vi "Count Event Message by Message.vi"(8 "error in (no error)":errorcluster, 9 "Timeout":i32, 10 "Message":string, 11 "Event Registration Refnum in":refnum<event-registration>) -> (0 "error out":errorcluster, 1 "Message Data":variant[](array[variant]), 2 "Count":i32, 3 "Event Registration Refnum out":refnum<event-registration>)   [LabVIEW 2020, in "Framework Test Support.lvlib" / "Event Helpers.lvlib"]
uses:
  Event Helpers.lvlib
  Framework/Process/Protected/Broadcasting/Broadcast Message Cluster.ctl
  Execution timer.vi
  Dequeue Event Message.vi
  Framework/Process/Process.lvclass
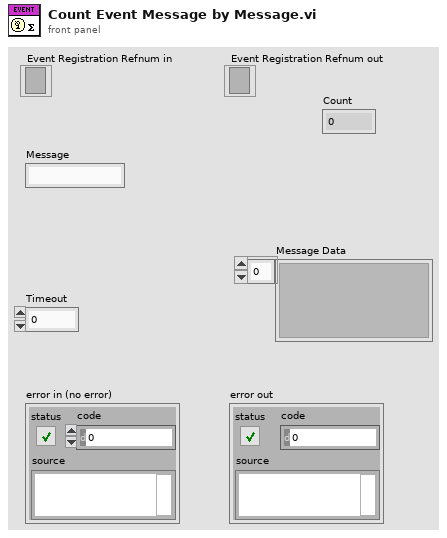
[diagram p1: front panel]
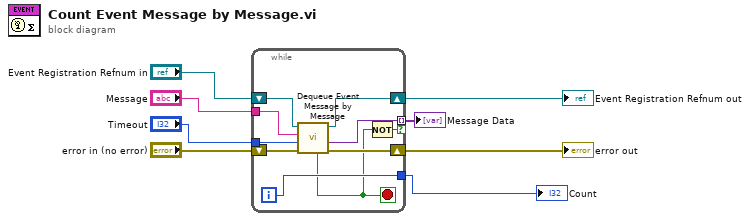
[diagram p0: block diagram]
diagram:
  n1 = while {
    tunnel: "Timeout" -> [w17]
    shift-right: [w18] -> w8
    shift-left: "error in (no error)" -> [w16]
    shift-right: [w15] -> w5
    shift-left: "Event Registration Refnum in" -> [w14]
    tunnel: "Message" -> [w13]
    tunnel: [w12] -> w2
    tunnel: [w11] -> w1 mode=indexing if=w9
    i -> [w12]
    stop <- w10 stop-if-true
    n2 = call "Dequeue Event Message by Message.vi"("error in (no error)"=w16, "Timeout (-1)"=w17, "Message"=w13, "Event Registration Refnum"=w14) -> ("error out"=w18:errorcluster, "Message Data"=w11:variant, "Event Registration Refnum Out"=w15:refnum<event-registration>, "Timed Out?"=w10:bool)  [unwired: 3 in, 1 out]
    n3 = Not(x=w10) -> (.not. x?=w9:bool)
  }
  "error out" <- w8
  "Event Registration Refnum out" <- w5
  "Count" <- w2
  "Message Data" <- w1
